vi "P3060_设置频率.vi"(8 "错误输入":errorcluster caption="错误输入（无错误）", 10 "频率":dbl, 11 "句柄输入":i32) -> (0 "错误输出":errorcluster, 2 "返回值":i32, 3 "句柄输出":i32)   [LabVIEW 2010]
doc: "发送异步通道数据"
uses:
  _SubVI/dll/P3060.dll
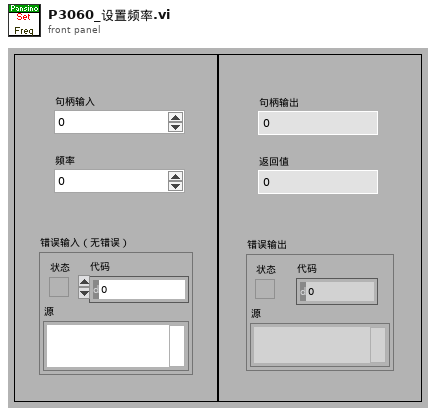
[diagram p1: front panel]
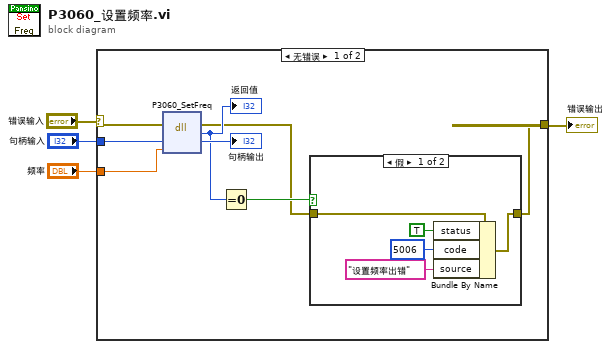
[diagram p0: block diagram]
diagram:
  n1 = case shown="无错误" "错误输入" {
    selector: "错误输入" -> [w12 w19]
    tunnel: [w6 w19] -> w3
    tunnel: "句柄输入" -> [w10 _]
    tunnel: "频率" -> [w5 _]
    frame No Error {
      n2 = dll-call lib="D:/driver/trunk/Drivers/P3060/P3060API/P3060APILV/Labview/P3060/_SubVI/dll/P3060.dll" fn="P3060_SetFreq"(error in=w12, "hDev"=w10, "FreqValue"=w5) -> (error out=w7:errorcluster, "return"=w9:i32, "hDev"=→"句柄输出":i32)  [unwired: 3 in, 1 out]
      "返回值" <- w9
      n3 = Equal To 0?(x=w9) -> (x = 0?=w8:bool)
      n4 = case shown="假" w8 {
        tunnel: [w16 w18] -> w6
        tunnel: w7 -> [w17 w18]
        frame False {
          n5 = Bundle By Name(cluster=w17, "status"=TRUE, "code"=5006, "source"="设置频率出错") -> (w16:errorcluster)
        }
        frame True {
        }
      }
    }
    frame Error {
    }
  }
  "错误输出" <- w3
